vi "NewWafer_Dial.vi"(2 "error in (no error)":errorcluster) -> (3 "Cancelled?":bool, 4 "Test Out":string(combo), 5 "Wafer ID Out":string, 6 "error out":errorcluster)   [LabVIEW 2012]
doc: "Use this template to create a dialog box with event handling."
panel:
  in  "Test":string(combo)="Initial"
  in  "Wafer ID":string
  in  "Cancel":bool
  in  "OK":bool
  # "Enter Wafer ID and Test Type"
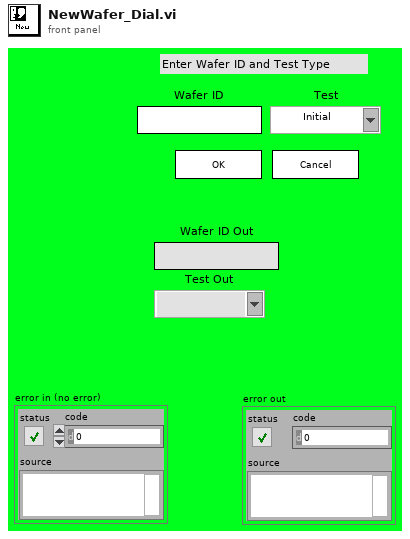
[diagram p1: front panel]
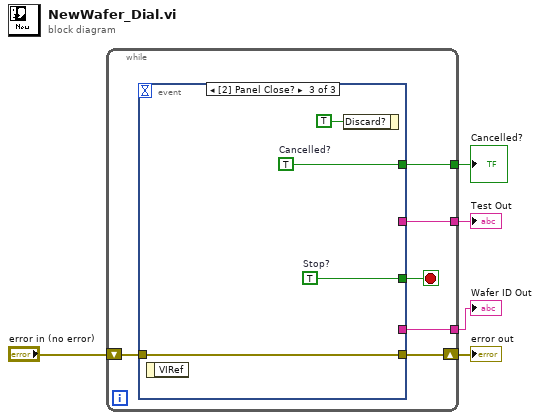
[diagram p0: block diagram]
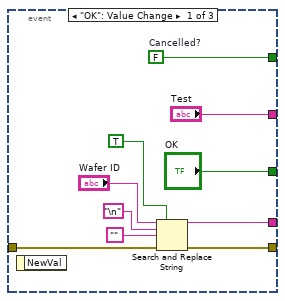
[diagram p2: hidden frame]
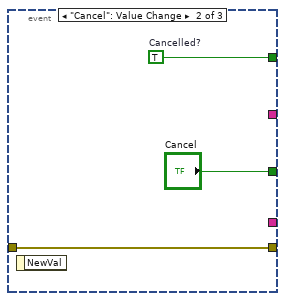
[diagram p3: hidden frame]
diagram:
  n1 = while {
    tunnel: [w10] -> w5
    tunnel: [w9] -> w4
    tunnel: [w8] -> w3
    shift-right: [w6] -> w2
    shift-left: "error in (no error)" -> [w7]
    stop <- w11 stop-if-true
    n2 = event shown="[2] Panel Close?" {
      selector: _ -> [_ _ _]
      dyn-events: _ -> [_ _ _]
      timeout: _ -> [_ _ _]
      tunnel: ["OK" "Cancel" w27] -> w11
      tunnel: [w21 w24 w26] -> w10
      tunnel: ["Test" _ _] -> w9
      tunnel: [w14 _ _] -> w8
      tunnel: w7 -> [w15 w22 w25]
      tunnel: [w12 w22 w25] -> w6
      event "OK": Value Change {
        w21 = FALSE  # Cancelled?
        n3 = event-data() -> ()  [unwired: 1 in, 1 out]
        n4 = Search and Replace String(replace all?=TRUE ("replace all? (F)"), input string="Wafer ID", search string="\n", replace string="", error in=w15) -> (result string=w14:string, error out=w12:errorcluster)  [unwired: 3 in, 2 out]
      }
      event "Cancel": Value Change {
        w24 = TRUE  # Cancelled?
        n5 = event-data() -> ()  [unwired: 1 in, 1 out]
      }
      event Panel Close? {
        w26 = TRUE  # Cancelled?
        w27 = TRUE  # Stop?
        n6 = event-data() -> ()  [unwired: 1 in, 1 out]
        n7 = event-data("Discard?"=TRUE) -> ()  [unwired: 1 in, 1 out]
      }
    }
  }
  "Cancelled?" <- w5
  "Wafer ID Out" <- w3
  "Test Out" <- w4
  "error out" <- w2
